vi "Filter Packets.vi"(8 "error in (no error)":errorcluster, 10 "CAN Data in":T1[](array[typedef]) {"Tags" format="%.0x"; "payload" format="%x"; "identifier" format="%x"}, 11 "CAN_Logic in":refnum<class "CAN_Logic.lvclass">) -> (0 "error out":errorcluster, 2 "CAN Data out":T1[](array[typedef]) {"Tags" format="%.0x"; "payload" format="%x"; "identifier" format="%x"}, 3 "CAN_Logic out":refnum<class "CAN_Logic.lvclass">)   [LabVIEW 2021, in "CAN_Logic.lvclass"]
uses:
  CAN_Logic.lvclass
  CAN_Logic.lvclass/CAN_Logic.ctl
  Channels/ChannelCommon/typedef/Datatype CAN.ctl
  Channels/ChannelCommon/ChannelCommon.lvlib
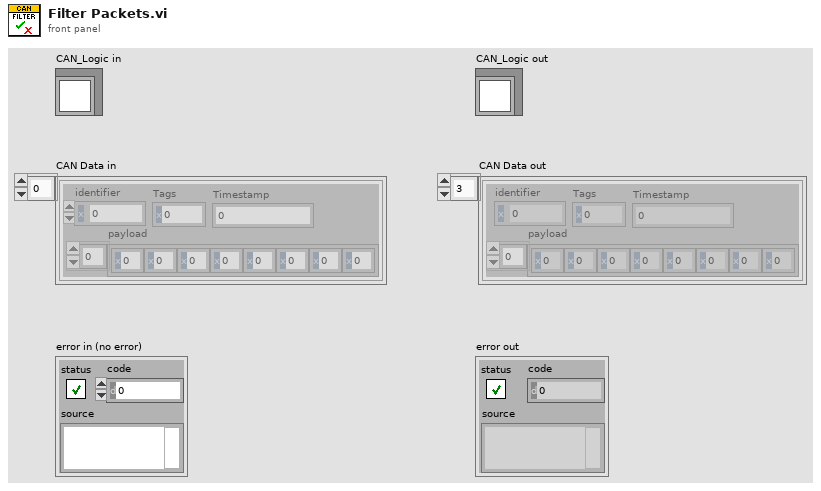
[diagram p1: front panel]
types:
  T1 = typedef "ChannelCommon.lvlib/Datatype CAN.ctl" = cluster{"payload":u8[], "identifier":u32, "Tags":u8, "Timestamp":u64}
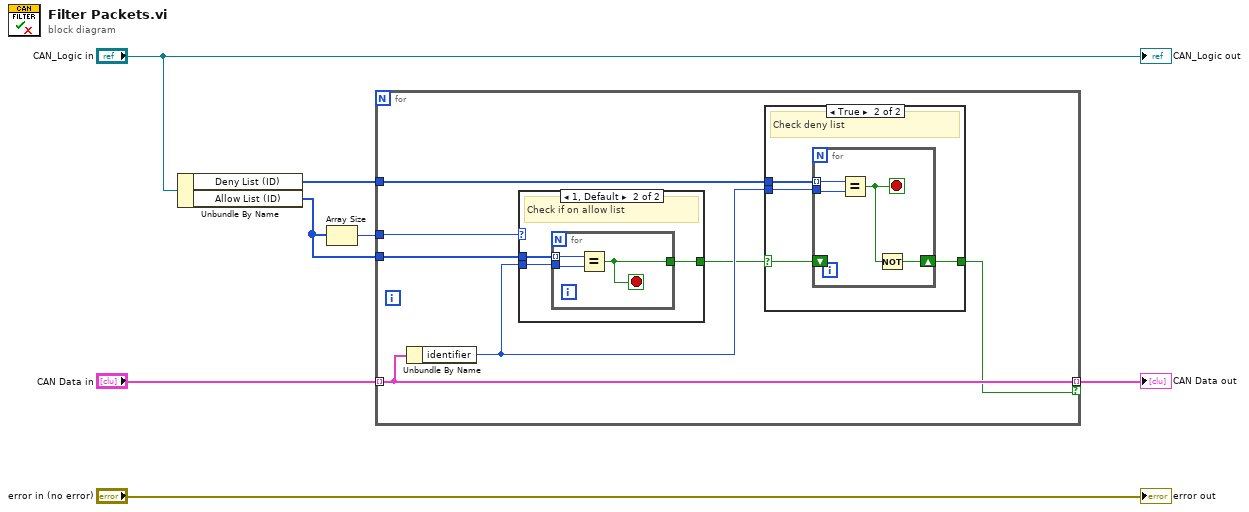
[diagram p0: block diagram]
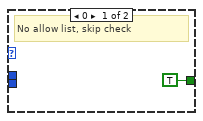
[diagram p3: hidden frame]
diagram:
  n1 = Unbundle By Name("CAN_Logic in") -> ("Deny List (ID)"=w4:u32[], "Allow List (ID)"=w3:u32[])
  n2 = Array Size(array=w3) -> (size(s)=w2:i32)
  n3 = for {
    tunnel: "CAN Data in" -> [w10] mode=indexing
    tunnel: w4 -> [w12]
    tunnel: w3 -> [w13]
    tunnel: w2 -> [w14]
    tunnel: [w10] -> w1 mode=indexing if=w9
    n4 = Unbundle By Name(w10) -> ("identifier"=w11:u32)
    n5 = case shown="1, Default" w14 {
      tunnel: w13 -> [_ w27]
      tunnel: w11 -> [_ w26]
      tunnel: [TRUE w25] -> w8
      frame 0 {
        # "No allow list, skip check"
      }
      frame 1, Default {
        # "Check if on allow list"
        n6 = for {
          tunnel: w27 -> [w29] mode=indexing
          tunnel: w26 -> [w30]
          tunnel: [w28] -> w25
          stop <- w28 stop-if-true
          n7 = Equal?(x=w29, y=w30) -> (x = y?=w28:bool)
        }
      }
    }
    n8 = case shown="True" w8 {
      selector: w8 -> [w15 w17]
      tunnel: w12 -> [_ w19]
      tunnel: w11 -> [_ w18]
      tunnel: [w15 w16] -> w9
      frame False {
        # "Failed allow list check, skip."
      }
      frame True {
        # "Check deny list"
        n9 = for {
          tunnel: w19 -> [w22] mode=indexing
          tunnel: w18 -> [w23]
          shift-right: [w20] -> w16
          shift-left: w17 -> [_]
          stop <- w21 stop-if-true
          n10 = Equal?(x=w22, y=w23) -> (x = y?=w21:bool)
          n11 = Not(x=w21) -> (.not. x?=w20:bool)
        }
      }
    }
  }
  "CAN Data out" <- w1
  "error out" <- "error in (no error)"
  "CAN_Logic out" <- "CAN_Logic in"
